vi "Newport ITX-D3N IBTHX Data.vi"(7 "Disable Filter?":bool=TRUE, 8 "error in (no error)":errorcluster, 11 "TCP Network Connection in":refnum<k5>) -> (0 "error out":errorcluster, 2 "iBTHX Data":T1, 3 "TCP Network Connection out":refnum<k5>)   [LabVIEW 2018]
uses:
  Type Definitions/iBTHX Data Values.ctl
  Type Definitions/iBTHX.ctl
panel:
  out "appended array":bool[](array[boolean])
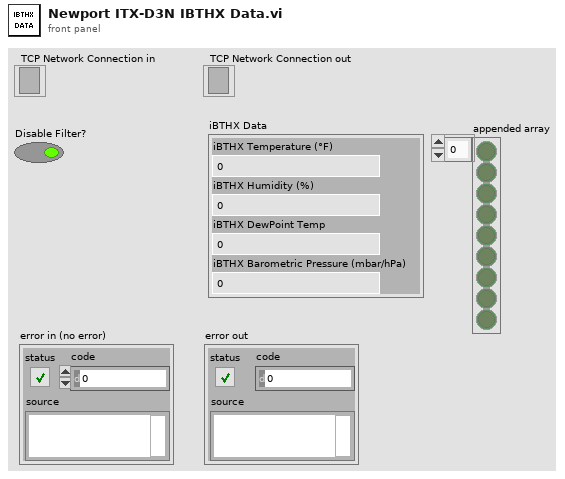
[diagram p1: front panel]
types:
  T1 = typedef "iBTHX Data Values.ctl" = cluster{"iBTHX Barometric Pressure (mbar/hPa)":dbl, "iBTHX Humidity (%)":dbl, "iBTHX Temperature (°F)":dbl, "iBTHX DewPoint Temp":dbl}
  T2 = typedef "iBTHX.ctl" = string
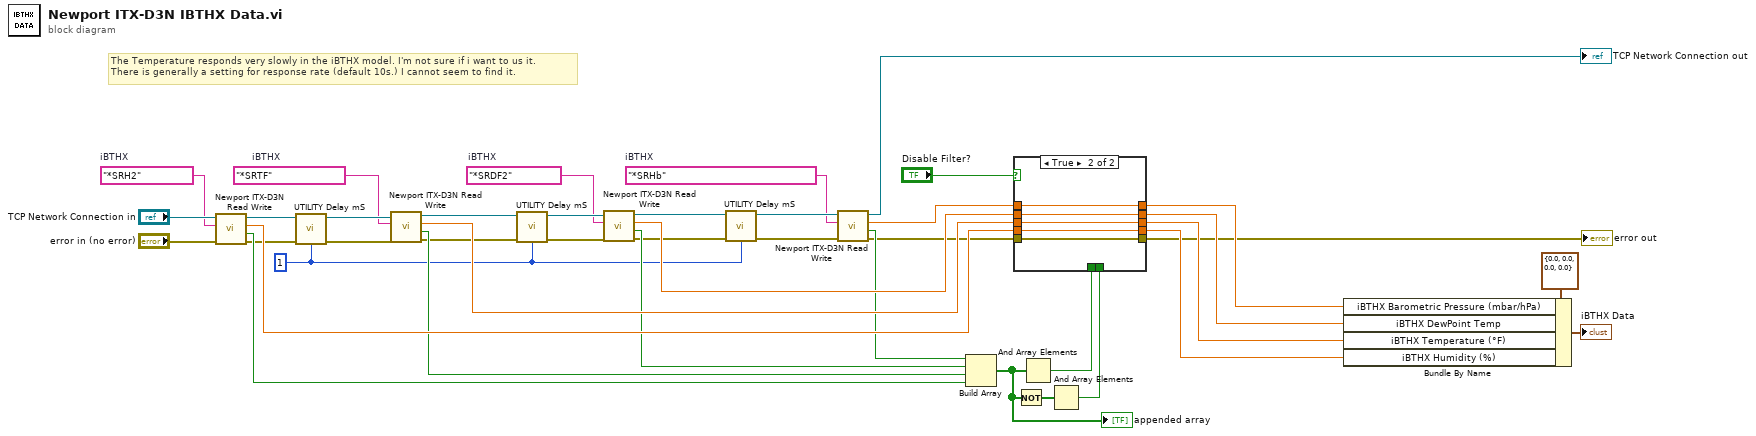
[diagram p0: block diagram]
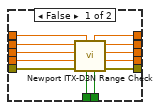
[diagram p2: hidden frame]
diagram:
  w5 = u32 1 ("milliseconds to wait")
  w33 = T2 "*SRDF2"  # iBTHX
  w32 = T2 "*SRTF"  # iBTHX
  w31 = T2 "*SRH2"  # iBTHX
  w30 = T2 "*SRHb"  # iBTHX
  # "The Temperature responds very slowly in the iBTHX model. I'm not sure if i want to us it.\nThere is generally a setting for response rate (default 10s.) I cannot seem to find it."
  n1 = call "Newport ITX-D3N Read Write.vi"("error in (no error)"="error in (no error)", "iTHX Commands"=w31, "TCP Network Connection in"="TCP Network Connection in") -> ("error out"=w11:errorcluster, "In Range?"=w14:bool, "Output Data"=w23:dbl, "TCP Network Connection out"=w35:refnum<k5>)  [unwired: 5 in]
  n2 = call "UTILITY Delay mS.vi"("Error In"=w11, "milliseconds to wait"=w5) -> ("Error Out"=w10:errorcluster)  [unwired: 13 in]
  n3 = call "Newport ITX-D3N Read Write.vi"("error in (no error)"=w10, "iTHX Commands"=w32, "TCP Network Connection in"=w35) -> ("error out"=w9:errorcluster, "In Range?"=w15:bool, "Output Data"=w24:dbl, "TCP Network Connection out"=w36:refnum<k5>)  [unwired: 5 in]
  n4 = call "UTILITY Delay mS.vi"("Error In"=w9, "milliseconds to wait"=w5) -> ("Error Out"=w8:errorcluster)  [unwired: 13 in]
  n5 = call "Newport ITX-D3N Read Write.vi"("error in (no error)"=w8, "iTHX Commands"=w33, "TCP Network Connection in"=w36) -> ("error out"=w7:errorcluster, "In Range?"=w16:bool, "Output Data"=w25:dbl, "TCP Network Connection out"=w37:refnum<k5>)  [unwired: 5 in]
  n6 = call "UTILITY Delay mS.vi"("Error In"=w7, "milliseconds to wait"=w5) -> ("Error Out"=w6:errorcluster)  [unwired: 13 in]
  n7 = call "Newport ITX-D3N Read Write.vi"("error in (no error)"=w6, "iTHX Commands"=w30, "TCP Network Connection in"=w37) -> ("error out"=w13:errorcluster, "In Range?"=w17:bool, "Output Data"=w19:dbl, "TCP Network Connection out"=→"TCP Network Connection out":refnum<k5>)  [unwired: 5 in]
  n8 = Build Array(w17, w16, w15, w14) -> (w3:bool[])
  "appended array" <- w3
  n9 = Not(x=w3) -> (.not. x?=w4:bool[])
  n10 = And Array Elements(Boolean array=w3) -> (logical AND=w26:bool)
  n11 = And Array Elements(Boolean array=w4) -> (logical AND=w2:bool)
  n12 = case shown="True" "Disable Filter?" {
    tunnel: w26 -> [w50 _]
    tunnel: w25 -> [w49 w54]
    tunnel: w24 -> [w48 w53]
    tunnel: w23 -> [w47 w52]
    tunnel: [w46 w54] -> w22
    tunnel: [w45 w53] -> w21
    tunnel: [w44 w52] -> w20
    tunnel: w19 -> [w43 w55]
    tunnel: [w42 w55] -> w18
    tunnel: w13 -> [w41 w51]
    tunnel: [w40 w51] -> w12
    tunnel: w2 -> [w39 _]
    frame False {
      n13 = call "Newport ITX-D3N Range Check.vi"("All Out of Range?"=w39, "In Range?"=w50, "Barometric Pressure"=w43, "Error In"=w41, "Humidity"=w47, "Temperature"=w48, "Dewpoint"=w49) -> ("Error Out"=w40:errorcluster, "Humidity Out"=w44:dbl, "Temperature Out"=w45:dbl, "Dewpoint Out"=w46:dbl, "Barometric Pressure Out"=w42:dbl)
    }
    frame True {
    }
  }
  "error out" <- w12
  n14 = Bundle By Name(cluster=T1 {"iBTHX Barometric Pressure (mbar/hPa)"=0.0, "iBTHX Humidity (%)"=0.0, "iBTHX Temperature (°F)"=0.0, "iBTHX DewPoint Temp"=0.0} ("iBTHX"), "iBTHX Barometric Pressure (mbar/hPa)"=w18, "iBTHX DewPoint Temp"=w22, "iBTHX Temperature (°F)"=w21, "iBTHX Humidity (%)"=w20) -> (→"iBTHX Data":T1)
